vi "Close Device Core.vi"(8 "error in (no error)":errorcluster, 11 "IVI_ACPwr in":refnum<class "IVI_ACPwr.lvclass">) -> (0 "error out":errorcluster, 3 "IVI_ACPwr out":refnum<class "IVI_ACPwr.lvclass">)   [LabVIEW 2015, in "IVI_ACPwr.lvlib" / "IVI_ACPwr.lvclass"]
doc: "Close device driver connection."
uses:
  IVI_ACPwr.lvclass
  IVI_ACPwr.lvclass/IVI_ACPwr.ctl
  CSPP_Core/Actors/CS++DeviceActor/CS++DeviceActor.lvclass
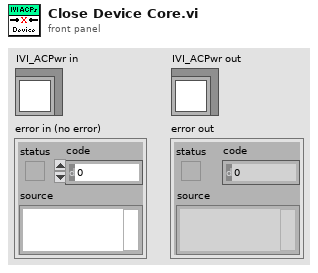
[diagram p1: front panel]
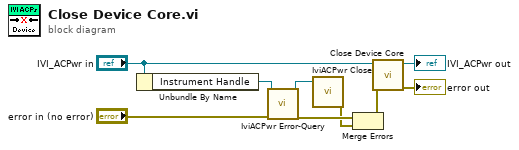
[diagram p0: block diagram]
diagram:
  n1 = Unbundle By Name("IVI_ACPwr in") -> ("Instrument Handle"=w6:refnum<k15>)
  n2 = call <vilib>:"IviACPwr Error-Query.vi"("error in (no error)"="error in (no error)", "instrument handle"=w6) -> ("error out"=w3:errorcluster, "instrument handle out"=w5:refnum<k15>)  [unwired: 6 in, 2 out]
  n3 = call <vilib>:"IviACPwr Close.vi"("instrument handle"=w5) -> ("error out"=w2:errorcluster)  [unwired: 10 in]
  n4 = Merge Errors(w3, w2) -> (w1:errorcluster)
  n5 = call-parent "Close Device Core.vi"("error in (no error)"=w1, "CS++DeviceActor in"="IVI_ACPwr in") -> ("error out"=→"error out":errorcluster, "CS++DeviceActor out"=→"IVI_ACPwr out":refnum<class "IVI_ACPwr.lvclass">)  [unwired: 8 in]
